vi "Move To Path.vi"(8 "error in (no error)":errorcluster, 10 "Paths":string[](array[string]), 11 "String":string) -> (0 "error out":errorcluster, 3 "String out":string)   [LabVIEW 2015, in "YAML Parser.lvclass"]
uses:
  YAML Parser.lvclass
  <vilib>/regexp/Match Regular Expression.xnode
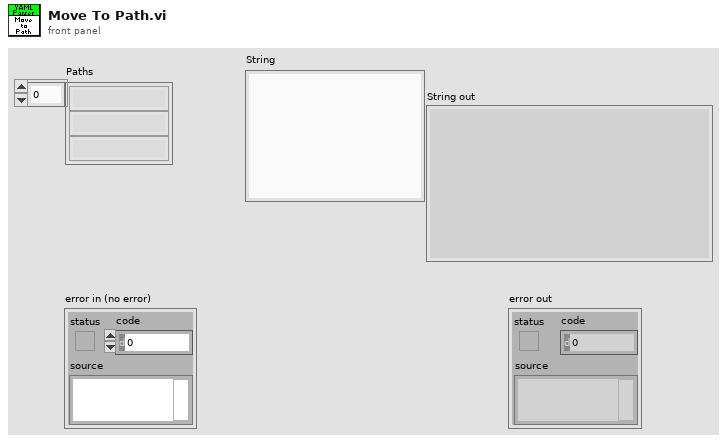
[diagram p1: front panel]
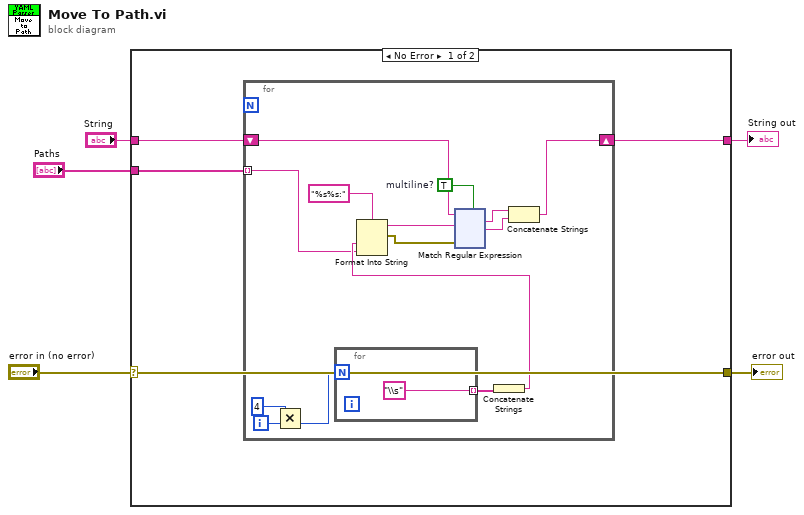
[diagram p0: block diagram]
diagram:
  n1 = case shown="No Error" "error in (no error)" {
    selector: "error in (no error)" -> [w9 w140]
    tunnel: [w9 w140] -> w4
    tunnel: "Paths" -> [w8 _]
    tunnel: "String" -> [w7 w139]
    tunnel: [w6 w139] -> w1
    frame No Error {
      n2 = for {
        tunnel: w8 -> [w14] mode=indexing
        shift-right: [w10] -> w6
        shift-left: w7 -> [w13]
        i -> [w19]
        w20 = TRUE  # multiline?
        n3 = Multiply(x=4, y=w19) -> (x*y=w17:i32)
        n4 = for {
          N: w17 -> [_]
          tunnel: ["\\s"] -> w18 mode=indexing
        }
        n5 = Concatenate Strings(w18) -> (w15:string)
        n6 = Format Into String(format string="%s%s:", w15, w14) -> (resulting string=w22:string, error out=w21:errorcluster)  [unwired: 2 in]
        n7 = xnode "Match Regular Expression"("input string"=w13, "regular expression"=w22, "error in"=w21, "multiline? (F)"=w20) -> ("whole match"=w12:string, "after match"=w11:string)  [unwired: 2 in, 3 out]
        n8 = Concatenate Strings(w12, w11) -> (w10:string)
      }
    }
    frame Error {
    }
  }
  "error out" <- w4
  "String out" <- w1
